vi "Clear.vi"(8 "error in (no error)":errorcluster, 11 "Execution UI In":refnum<class "Execution UI.lvclass">) -> (0 "error out":errorcluster, 3 "Execution UI Out":refnum<class "Execution UI.lvclass">)   [LabVIEW 2020, in "Execution UI.lvclass"]
uses:
  Execution UI.lvclass
  Execution UI.lvclass/Execution UI.ctl
  Application Framework/Process Classes/Process/Process.lvclass
  Test Runner/Test Runner.lvclass
  Report Generator/Report Generator.lvclass
  Icon Decorator/Icon Decorator.lvclass
  Execution Profiler/Execution Profiler.lvclass
  Application Framework/Process Classes/Error Handler/Error Handler.lvclass
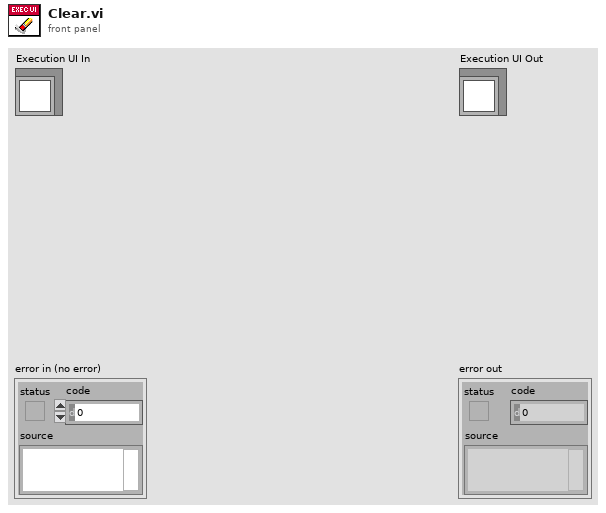
[diagram p1: front panel]
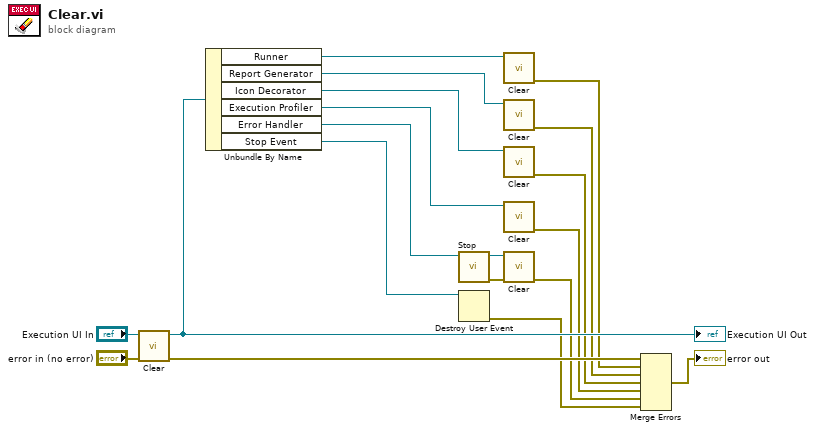
[diagram p0: block diagram]
diagram:
  n1 = call-parent "Clear.vi"("error in (no error)"="error in (no error)", "Process In"="Execution UI In") -> ("error out"=w19:errorcluster, "Process Out"=w14:refnum<class "Execution UI.lvclass">)  [unwired: 8 in]
  "Execution UI Out" <- w14
  n2 = Unbundle By Name(w14) -> ("Runner"=w15:refnum<class "Test Runner.lvclass">, "Report Generator"=w16:refnum<class "Report Generator.lvclass">, "Icon Decorator"=w10:refnum<class "Icon Decorator.lvclass">, "Execution Profiler"=w8:refnum<class "Execution Profiler.lvclass">, "Error Handler"=w4:refnum<class "Error Handler.lvclass">, "Stop Event"=w3:refnum<user-event>)
  n3 = call-dynamic "Stop.vi"("Process In"=w4) -> ("error out"=w5:errorcluster, "Process Out"=w6:refnum<class "Error Handler.lvclass">)  [unwired: 8 in, 1 out]
  n4 = Destroy User Event(user event=w3) -> (error out=w1:errorcluster)  [unwired: 1 in]
  n5 = call-dynamic "Clear.vi"("Test Runner In"=w15) -> ("error out"=w12:errorcluster)  [unwired: 9 in, 1 out]
  n6 = call-dynamic "Clear.vi"("Process In"=w16) -> ("error out"=w11:errorcluster)  [unwired: 9 in, 1 out]
  n7 = call-dynamic "Clear.vi"("Process In"=w10) -> ("error out"=w9:errorcluster)  [unwired: 9 in, 1 out]
  n8 = call-dynamic "Clear.vi"("Process In"=w8) -> ("error out"=w7:errorcluster)  [unwired: 9 in, 1 out]
  n9 = call-dynamic "Clear.vi"("error in (no error)"=w5, "Error Handler In"=w6) -> ("error out"=w2:errorcluster)  [unwired: 8 in, 1 out]
  n10 = Merge Errors(w19, w12, w11, w9, w7, w2, w1) -> (→"error out":errorcluster)
